vi "Enforce Robot Rules.vi"(5 "max V":dbl, 6 "Drive Type":T1=enum."Holonomic", 7 "Overrides":T2 {"Angle Override" step=5.0; "Velocity Override" step=5.0; "Angular Override" step=5.0}, 8 "turn accel":dbl, 9 "Disable":bool, 10 "New Points":cluster{"x":dbl, "y":dbl, "th":dbl}[](array[cluster]), 11 "Original Points":cluster{"x":dbl, "y":dbl, "th":dbl}[](array[cluster])) -> (2 "Overrides Out":T2 {"Angle Override" step=5.0; "Velocity Override" step=5.0; "Angular Override" step=5.0}, 3 "Points out":cluster{"x":dbl, "y":dbl, "th":dbl}[](array[cluster]))   [LabVIEW 2025]
uses:
  Types/Overrides.ctl
  Types/Drive Type.ctl
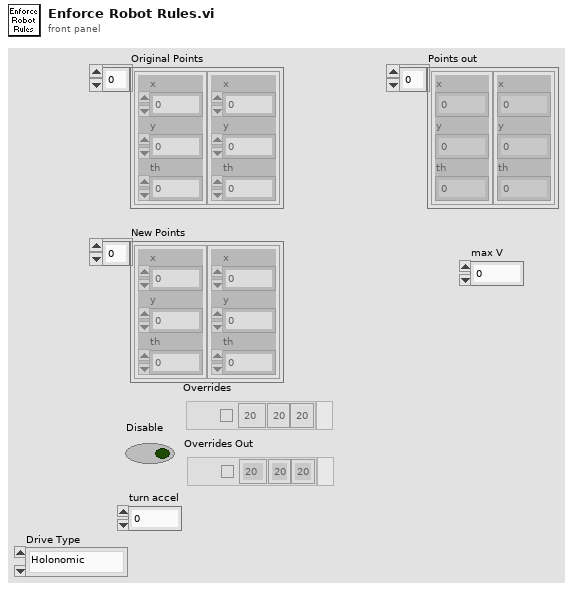
[diagram p1: front panel]
types:
  T1 = typedef "Drive Type.ctl" = enum16{"Nonholonomic", "Holonomic"}
  T2 = typedef "Overrides.ctl" = cluster{"Count":string, "Angular Override":dbl, "Enabled?":bool, "Velocity Override":dbl, "Angle Override":dbl}[]
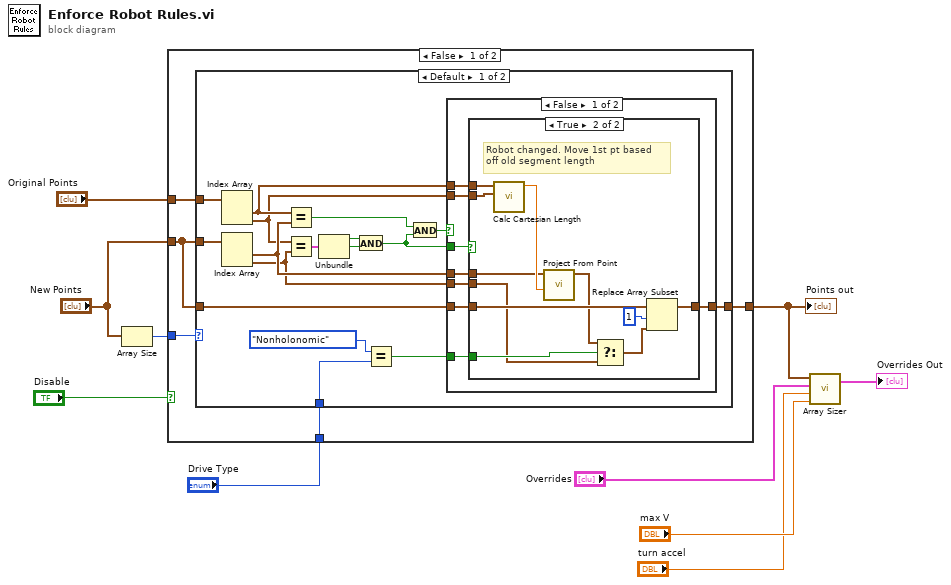
[diagram p0: block diagram]
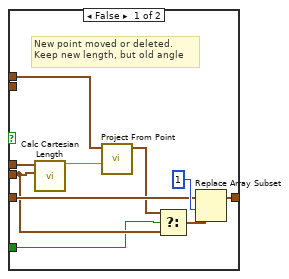
[diagram p2: hidden frame]
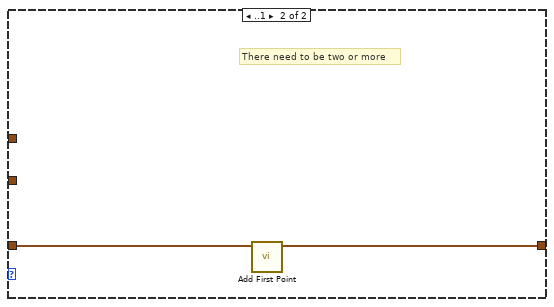
[diagram p4: hidden frame]
diagram:
  n1 = Array Size(array="New Points") -> (size(s)=w9:i32)
  n2 = case shown="False" "Disable" {
    tunnel: "Original Points" -> [w15 _]
    tunnel: w9 -> [w14 _]
    tunnel: [w13 w65] -> w6
    tunnel: "New Points" -> [w12 w65]
    tunnel: "Drive Type" -> [w11 _]
    frame False {
      n3 = case shown="Default" w14 {
        tunnel: w15 -> [w32 _]
        tunnel: w12 -> [w31 _]
        tunnel: [w29 w64] -> w13
        tunnel: w12 -> [w28 w63]
        tunnel: w11 -> [w18 _]
        frame Default {
          n4 = Index Array(array=w32) -> (element #1=w26:cluster{"x":dbl, "y":dbl, "th":dbl}, element #2=w23:cluster{"x":dbl, "y":dbl, "th":dbl})  [unwired: 2 in]
          n5 = Index Array(array=w31) -> (element #1=w25:cluster{"x":dbl, "y":dbl, "th":dbl}, element #2=w24:cluster{"x":dbl, "y":dbl, "th":dbl})  [unwired: 2 in]
          n6 = Equal?(x=w26, y=w25) -> (x = y?=w27:bool)
          n7 = Equal?(x=w23, y=w24) -> (x = y?=w22:cluster{"x":bool, "y":bool, "th":bool})
          n8 = Unbundle(w22) -> ("x"=w21:bool, "y"=w20:bool)  [unwired: 1 out]
          n9 = And(x=w21, y=w20) -> (x .and. y?=w19:bool)
          n10 = Equal?(x=Drive_Type."Nonholonomic" ("Drive Type"), y=w18) -> (x = y?=w16:bool)
          n11 = And(x=w27, y=w19) -> (x .and. y?=w30:bool)
          n12 = case shown="False" w30 {
            tunnel: [w36 w62] -> w29
            tunnel: w28 -> [w34 w62]
            tunnel: w19 -> [w38 _]
            tunnel: w26 -> [w40 _]
            tunnel: w23 -> [w39 _]
            tunnel: w25 -> [w37 _]
            tunnel: w24 -> [w35 _]
            tunnel: w16 -> [w33 _]
            frame False {
              n13 = case shown="True" w38 {
                tunnel: w40 -> [w46 w61]
                tunnel: w39 -> [_ w60]
                tunnel: w37 -> [w50 w55]
                tunnel: [w47 w58] -> w36
                tunnel: w35 -> [w43 w52]
                tunnel: w34 -> [w48 w59]
                tunnel: w33 -> [w41 w54]
                frame False {
                  # "New point moved or deleted.\nKeep new length, but old angle"
                  n14 = call "Calc Cartesian Length.vi"("Point 2"=w43, "Point 1"=w50) -> ("Length (f)"=w45:dbl)  [unwired: 8 in, 1 out]
                  n15 = call "Project From Point.vi"("distance"=w45, "Point In"=w46) -> ("Point Out"=w44:cluster{"x":dbl, "y":dbl, "th":dbl})  [unwired: 9 in]
                  n16 = Select(t=w44, s=w41, f=w43) -> (s? t:f=w42:cluster{"x":dbl, "y":dbl, "th":dbl})
                  n17 = Replace Array Subset(array=w48, new element=w42, index=1) -> (w47:cluster{"x":dbl, "y":dbl, "th":dbl}[])
                }
                frame True {
                  # "Robot changed. Move 1st pt based\noff old segment length"
                  n18 = call "Calc Cartesian Length.vi"("Point 2"=w60, "Point 1"=w61) -> ("Length (f)"=w56:dbl)  [unwired: 8 in, 1 out]
                  n19 = call "Project From Point.vi"("distance"=w56, "Point In"=w55) -> ("Point Out"=w53:cluster{"x":dbl, "y":dbl, "th":dbl})  [unwired: 9 in]
                  n20 = Select(t=w53, s=w54, f=w52) -> (s? t:f=w51:cluster{"x":dbl, "y":dbl, "th":dbl})
                  n21 = Replace Array Subset(array=w59, new element=w51, index=1) -> (w58:cluster{"x":dbl, "y":dbl, "th":dbl}[])
                }
              }
            }
            frame True {
              # "First two elements didn't\nchange. assume they are\ngood"
            }
          }
        }
        frame ..1 {
          # "There need to be two or more"
          n22 = call "Add First Point.vi"("Initial Points"=w63) -> ("Points"=w64:cluster{"x":dbl, "y":dbl, "th":dbl}[])  [unwired: 10 in]
        }
      }
    }
    frame True {
    }
  }
  "Points out" <- w6
  n23 = call "Array Sizer.vi"("maxV"="max V", "turn accel"="turn accel", "Overrides"="Overrides", "Points out"=w6) -> ("Overrides out"=→"Overrides Out":T2)  [unwired: 1 in]
